vi "Day 18 Universal gate.vi"() -> ()   [LabVIEW 2026]
panel:
  out "NAND-NOT Grid":bool[][](array[boolean])
  out "NAND-OR Grid":bool[][](array[boolean])
  out "NAND-AND Grid":bool[][](array[boolean])
  out "NOR-AND Grid":bool[][](array[boolean])
  out "NOR-OR Grid":bool[][](array[boolean])
  out "NOR-NOT Grid":bool[][](array[boolean])
  out "NOR VERIFICATION GRID":bool[][](array[boolean])
  # "Building Logic Gates with NAND & NOR"
  # "NOR VERIFICATION GRID"
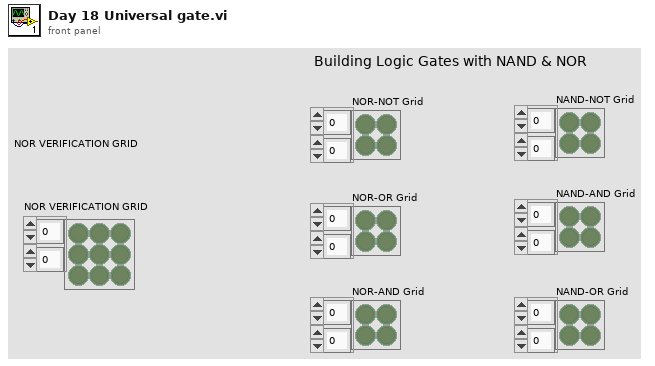
[diagram p1: front panel]
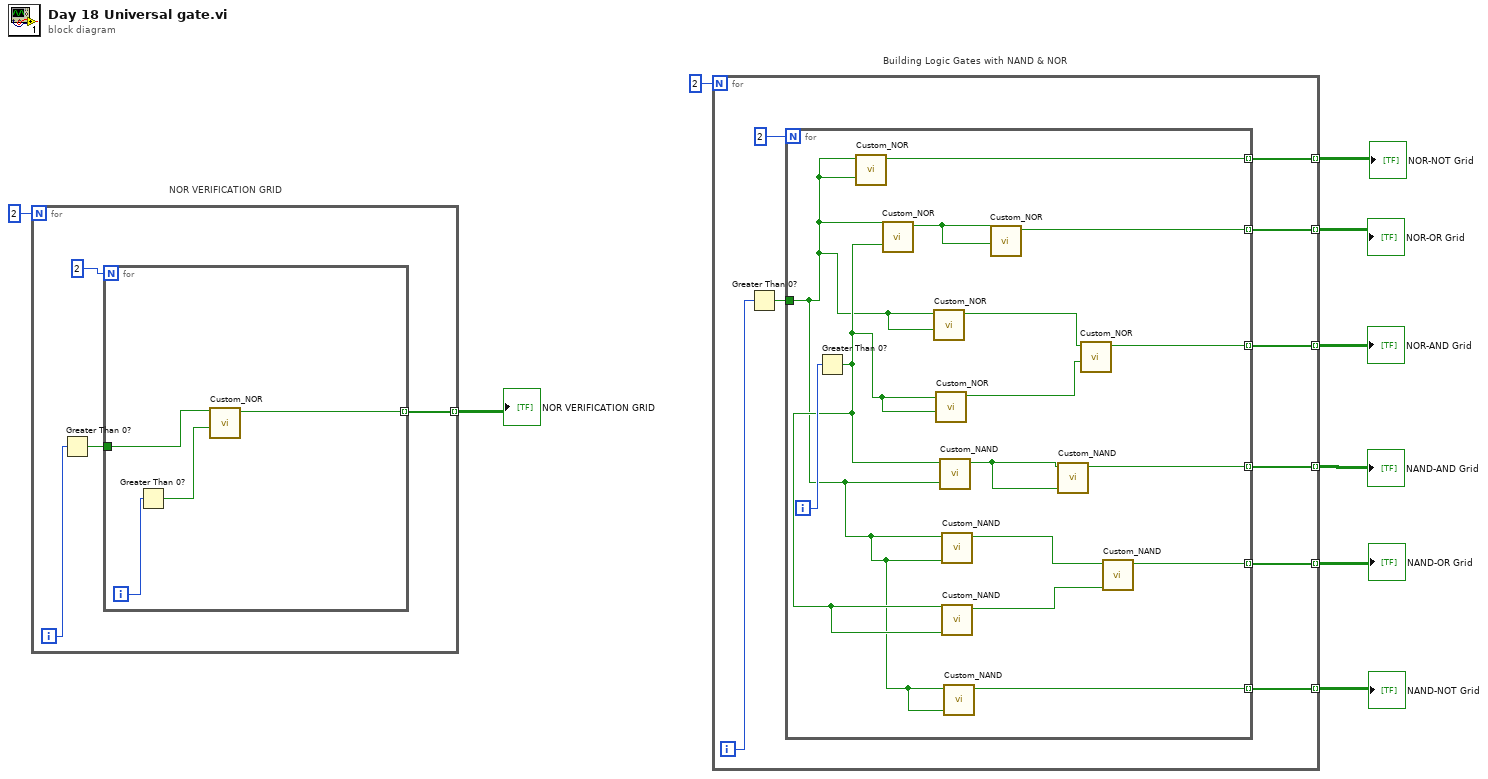
[diagram p0: block diagram]
diagram:
  # "NOR VERIFICATION GRID"
  # "Building Logic Gates with NAND & NOR"
  n1 = for {
    N: 2 -> [_]
    tunnel: [w10] -> w8 mode=indexing
    i -> [w12]
    n2 = Greater Than 0?(x=w12) -> (x > 0?=w11:bool)
    n3 = for {
      N: 2 -> [_]
      tunnel: w11 -> [w15]
      tunnel: [w14] -> w10 mode=indexing
      i -> [w17]
      n4 = Greater Than 0?(x=w17) -> (x > 0?=w16:bool)
      n5 = call "Custom_NOR.vi"("Input B"=w16, "Input A"=w15) -> ("Output Y"=w14:bool)  [unwired: 9 in]
    }
  }
  "NOR VERIFICATION GRID" <- w8
  n6 = for {
    N: 2 -> [_]
    tunnel: [w23] -> w6 mode=indexing
    tunnel: [w22] -> w5 mode=indexing
    tunnel: [w21] -> w4 mode=indexing
    tunnel: [w20] -> w3 mode=indexing
    tunnel: [w19] -> w2 mode=indexing
    tunnel: [w18] -> w1 mode=indexing
    i -> [w25]
    n7 = Greater Than 0?(x=w25) -> (x > 0?=w24:bool)
    n8 = for {
      N: 2 -> [_]
      tunnel: w24 -> [w28]
      tunnel: [w33] -> w23 mode=indexing
      tunnel: [w32] -> w22 mode=indexing
      tunnel: [w31] -> w21 mode=indexing
      tunnel: [w30] -> w20 mode=indexing
      tunnel: [w29] -> w19 mode=indexing
      tunnel: [w27] -> w18 mode=indexing
      i -> [w41]
      n9 = Greater Than 0?(x=w41) -> (x > 0?=w36:bool)
      n10 = call "Custom_NOR.vi"("Input B"=w28, "Input A"=w28) -> ("Output Y"=w33:bool)  [unwired: 9 in]
      n11 = call "Custom_NOR.vi"("Input B"=w36, "Input A"=w28) -> ("Output Y"=w40:bool)  [unwired: 9 in]
      n12 = call "Custom_NOR.vi"("Input B"=w28, "Input A"=w28) -> ("Output Y"=w39:bool)  [unwired: 9 in]
      n13 = call "Custom_NOR.vi"("Input B"=w36, "Input A"=w36) -> ("Output Y"=w38:bool)  [unwired: 9 in]
      n14 = call "Custom_NAND.vi"("Input B"=w28, "Input A"=w36) -> ("Output"=w37:bool)  [unwired: 9 in]
      n15 = call "Custom_NAND.vi"("Input B"=w28, "Input A"=w28) -> ("Output"=w35:bool)  [unwired: 9 in]
      n16 = call "Custom_NAND.vi"("Input B"=w36, "Input A"=w36) -> ("Output"=w34:bool)  [unwired: 9 in]
      n17 = call "Custom_NAND.vi"("Input B"=w28, "Input A"=w28) -> ("Output"=w27:bool)  [unwired: 9 in]
      n18 = call "Custom_NOR.vi"("Input B"=w40, "Input A"=w40) -> ("Output Y"=w32:bool)  [unwired: 9 in]
      n19 = call "Custom_NAND.vi"("Input B"=w37, "Input A"=w37) -> ("Output"=w30:bool)  [unwired: 9 in]
      n20 = call "Custom_NOR.vi"("Input B"=w38, "Input A"=w39) -> ("Output Y"=w31:bool)  [unwired: 9 in]
      n21 = call "Custom_NAND.vi"("Input B"=w34, "Input A"=w35) -> ("Output"=w29:bool)  [unwired: 9 in]
    }
  }
  "NOR-NOT Grid" <- w6
  "NOR-OR Grid" <- w5
  "NOR-AND Grid" <- w4
  "NAND-AND Grid" <- w3
  "NAND-OR Grid" <- w2
  "NAND-NOT Grid" <- w1
